vi "Power Spectrum.vi"(8 "error in":errorcluster, 9 "sample rate":dbl=100000000.0, 10 "scaling factor":dbl=3.0517578125e-05, 11 "ai data":i16[](array[numeric])) -> (0 "error out":errorcluster, 3 "magnitude":cluster{"f0":dbl, "df":dbl, "magnitude":dbl[]} {"magnitude" format="%.2p"; "f0" format="%0.2p"; "df" format="%0.2p"})   [LabVIEW 2018, in "Lock-In Amplifier Example Host.lvlib"]
uses:
  Lock-In Amplifier Example Host.lvlib
  <vilib>/measure/maspectr.llb/FFT Spectrum (Mag-Phase) for 1 Chan.vi
  <vilib>/measure/NI_MAPro.lvlib
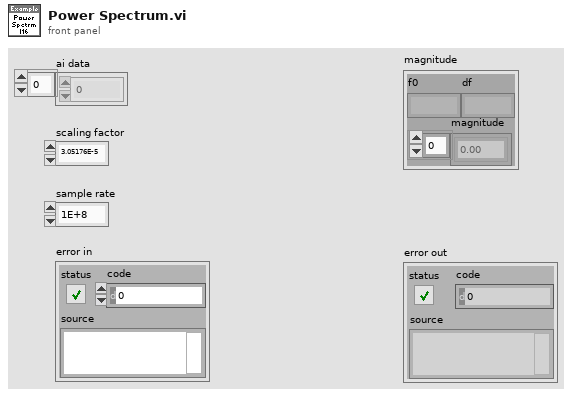
[diagram p1: front panel]
types:
  T1 = cluster{"dB On (F)":bool, "unwrap phase (F)":bool, "convert to degree (F)":bool}
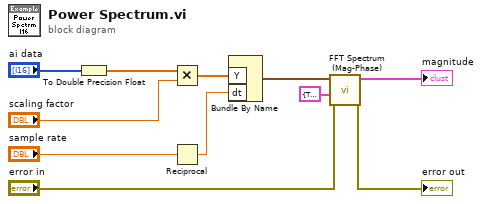
[diagram p0: block diagram]
diagram:
  n1 = To Double Precision Float(number="ai data") -> (double precision float=w10:dbl[])
  n2 = Multiply(x=w10, y="scaling factor") -> (x*y=w8:dbl[])
  n3 = Reciprocal(x="sample rate") -> (1/x=w1:dbl)
  n4 = Bundle By Name("Y"=w8, "dt"=w1) -> (w6:waveform(dbl))  [unwired: 1 in]
  n5 = call-poly <vilib>:"FFT Spectrum (Mag-Phase).vi"("error in (no error)"="error in", "view"=T1 {"dB On (F)"=TRUE, "unwrap phase (F)"=FALSE, "convert to degree (F)"=FALSE}, "time signal"=w6) -> ("error out"=→"error out":errorcluster, "magnitude"=→"magnitude":cluster{"f0":dbl, "df":dbl, "magnitude":dbl[]})  [unwired: 4 in, 3 out]
